vi "unlock_lvclass_ctl.vi"(8 "error in (no error)":errorcluster, 11 "Flattened\nPrivateDataCTL line":string) -> (0 "error out":errorcluster, 3 "Unlocked Flattened CTL line":string)   [LabVIEW 2020]
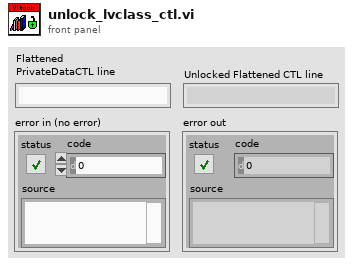
[diagram p1: front panel]
types:
  T1 = map{string, cluster{"Offset":i32, "Data":string}}
  T2 = cluster{"version":u32, "Flags":u32, "viFlags2":u32, "viFlags0C":u32, "viFlags10":u32, "buttonsHidden":u16, "frontpFlags":u16, "instrState":u32, "execState":u32, "execPrio":u16, "viType":u16, "prefExecSyst":i32, "field28":u32, "field2C":u32, "field30":u32, "viSignatureHi":u64, "viSignatureLo":u64, "alignGridFP":u32, "alignGridBD":u32, "field4C":u16, "ctrlIndStyle":u16, "field50_md5Hi":u64, "field50_md5Lo":u64, "libHi":u64, "libLo":u64}
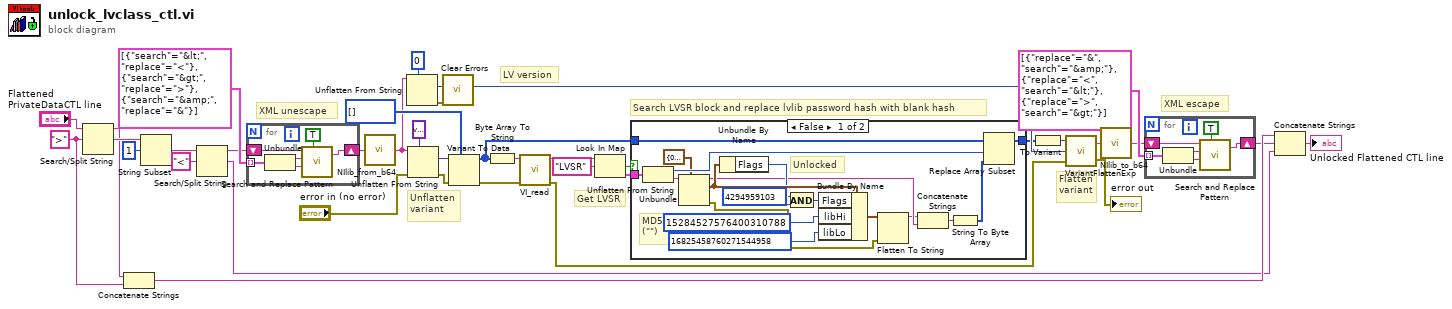
[diagram p0: block diagram]
diagram:
  w21 = ">" ("search string/char (-)")
  # "Get LVSR"
  # "XML escape"
  # "Search LVSR block and replace lvlib password hash with blank hash"
  # "Flatten\nvariant"
  # "LV version"
  # "Unflatten\nvariant"
  # "XML unescape"
  n1 = Search/Split String(string="Flattened\nPrivateDataCTL line", search string/char (-)=w21) -> (substring before match=w22:string, match + rest of string=w24:string)  [unwired: 1 in, 1 out]
  n2 = Concatenate Strings(w22, w21) -> (w16:string)
  n3 = String Subset(string=w24, offset (0)=1) -> (substring=w19:string)  [unwired: 1 in]
  n4 = Search/Split String(string=w19, search string/char (-)="<") -> (substring before match=w17:string, match + rest of string=w14:string)  [unwired: 1 in, 1 out]
  n5 = for {
    shift-right: [w38] -> w9
    shift-left: w17 -> [w43]
    tunnel: cluster{"search":string, "replace":string}[] [{"search"="&lt;", "replace"="<"}, {"search"="&gt;", "replace"=">"}, {"search"="&amp;", "replace"="&"}] -> [w41] mode=indexing
    n6 = Unbundle(w41) -> ("search"=w40:string, "replace"=w39:string)
    n7 = call <vilib>:"Search and Replace Pattern.vi"("string"=w43, "regular expression (\"\")"=w40, "replace string (\"\")"=w39, "replace all? (F)"=TRUE) -> ("result string"=w38:string)  [unwired: 1 in, 1 out]
  }
  n8 = call "NIlib_from_b64.vi"("base64 in"=w9) -> ("string out"=w8:string)
  n9 = Unflatten From String(type=u32 0, binary string=w8) -> (value=w31:u32, error out=w5:errorcluster)  [unwired: 3 in, 1 out]
  n10 = Unflatten From String(type=variant ("variant"), binary string=w8, error in (no error)="error in (no error)") -> (value=w34:variant, error out=w35:errorcluster)  [unwired: 2 in, 1 out]
  n11 = call <vilib>:"Clear Errors.vi"("error in (no error)"=w5) -> ()  [unwired: 5 in, 2 out]
  n12 = Variant To Data(error in=w35, type=u8[] [], Variant=w34) -> (data=w26:u8[], error out=w7:errorcluster)
  n13 = Byte Array To String(unsigned byte array=w26) -> (string=w12:string)
  n14 = call "VI_read.vi"("error in (no error)"=w7, "File bytestream"=w12) -> ("error out"=w6:errorcluster, "Blocks"=w3:T1)  [unwired: 5 in, 3 out]
  n15 = Look In Map(map=w3, key="LVSR") -> (key not found?=w2:bool, value=w1:cluster{"Offset":i32, "Data":string})  [unwired: 1 in]
  n16 = case shown="False" w2 {
    tunnel: w26 -> [w45 w62]
    tunnel: w1 -> [w46 _]
    tunnel: [w44 w62] -> w25
    frame False {
      # "MD5\n(\"\")"
      # "Unlocked"
      n17 = Unbundle(w46) -> ("Offset"=w61:i32, "Data"=w55:string)
      n18 = Unflatten From String(type=T2 {"version"=0, "Flags"=0, "viFlags2"=0, "viFlags0C"=0, "viFlags10"=0, "buttonsHidden"=0, "frontpFlags"=0, "instrState"=0, "execState"=0, "execPrio"=0, "viType"=0, "prefExecSyst"=0, "field28"=0, "field2C"=0, "field30"=0, "viSignatureHi"=0, "viSignatureLo"=0, "alignGridFP"=0, "alignGridBD"=0, "field4C"=0, "ctrlIndStyle"=0, "field50_md5Hi"=0, "field50_md5Lo"=0, "libHi"=0, "libLo"=0} ("LVSR"), binary string=w55) -> (rest of the binary string=w48:string, value=w57:T2, error out=w58:errorcluster)  [unwired: 3 in]
      n19 = Unbundle By Name(w57) -> ("Flags"=w56:u32)
      n20 = And(x=u32 4294959103 ("Unlocked"), y=w56) -> (x .and. y?=w54:u32)
      n21 = Bundle By Name(cluster=w57, "Flags"=w54, "libHi"=u64 15284527576400310788 ("libpass_md5Hi"), "libLo"=u64 16825458760271544958 ("libpass_md5Lo")) -> (w49:T2)
      n22 = Flatten To String(anything=w49, error in (no error)=w58) -> (data string=w47:string)  [unwired: 2 in, 2 out]
      n23 = Concatenate Strings(w47, w48) -> (w60:string)
      n24 = String To Byte Array(string=w60) -> (unsigned byte array=w59:u8[])
      n25 = Replace Array Subset(array=w45, new element=w59, index=w61) -> (w44:u8[])
    }
    frame True {
      # "No LVSR block!"
    }
  }
  n26 = To Variant(anything=w25) -> (Variant=w30:variant)
  n27 = call <vilib>:"VariantFlattenExp.vi"("error in (no error)"=w6, "version"=w31, "variant"=w30) -> ("error out"=→"error out":errorcluster, "data string"=w11:string)
  n28 = call "NIlib_to_b64.vi"("string in"=w11) -> ("base64 out"=w10:string)
  n29 = for {
    shift-right: [w63] -> w15
    shift-left: w10 -> [w68]
    tunnel: cluster{"replace":string, "search":string}[] [{"replace"="&", "search"="&amp;"}, {"replace"="<", "search"="&lt;"}, {"replace"=">", "search"="&gt;"}] -> [w66] mode=indexing
    n30 = Unbundle(w66) -> ("replace"=w65:string, "search"=w64:string)
    n31 = call <vilib>:"Search and Replace Pattern.vi"("string"=w68, "regular expression (\"\")"=w65, "replace string (\"\")"=w64, "replace all? (F)"=TRUE) -> ("result string"=w63:string)  [unwired: 1 in, 1 out]
  }
  n32 = Concatenate Strings(w16, w15, w14) -> (→"Unlocked Flattened CTL line":string)
